vi "element A-D.vi"(8 "error in (no error)":errorcluster) -> (0 "error out":errorcluster, 3 "max(x,y)":i64)   [LabVIEW 2020, in "Settings.lvlib"]
uses:
  Settings.lvlib
  <vilib>/drjdpowell/SQLite Library/SQL Connection/Open (path).vi
  <vilib>/drjdpowell/SQLite Library/SQL Connection/Open (string).vi
  <vilib>/AdvancedString/Path To Command Line String.vi
  <vilib>/drjdpowell/SQLite Library/SQL Connection/Execute SQL (1D Integer results).vi
  <vilib>/drjdpowell/SQLite Library/SQL Connection/Connection.lvclass
  <vilib>/drjdpowell/SQLite Library/SQLite.lvlib
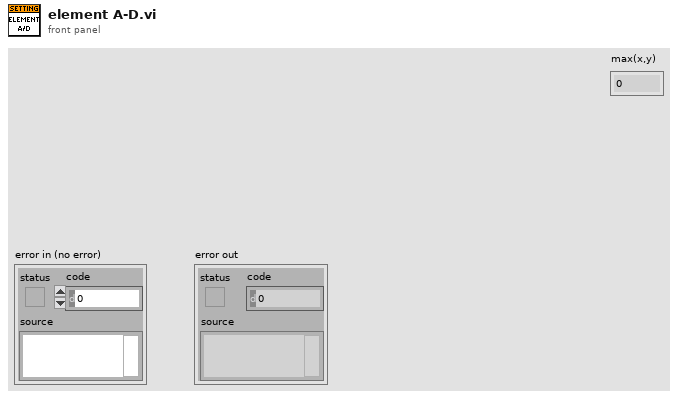
[diagram p1: front panel]
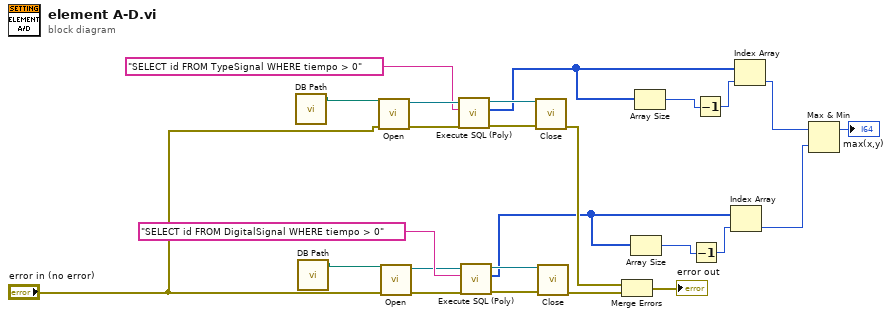
[diagram p0: block diagram]
diagram:
  n1 = call "DB Path.vi"() -> ("DB path"=w20:path)  [unwired: 11 in]
  n2 = call "DB Path.vi"() -> ("DB path"=w18:path)  [unwired: 11 in]
  n3 = call-poly <vilib>:"Open.vi"("error in (no error)"="error in (no error)", "db file"=w20) -> ("error out"=w24:errorcluster, "SQLite Connection"=w23:refnum<class "Connection.lvclass">)  [unwired: 8 in]
  n4 = call-poly <vilib>:"Open.vi"("error in (no error)"="error in (no error)", "db file"=w18) -> ("error out"=w13:errorcluster, "SQLite Connection"=w14:refnum<class "Connection.lvclass">)  [unwired: 8 in]
  n5 = call-poly <vilib>:"Execute SQL (Poly).vi"("error in (no error)"=w24, "SQL"="SELECT id FROM TypeSignal WHERE tiempo > 0", "SQLite Connection in"=w23) -> ("error out"=w21:errorcluster, "Result Set"=w9:i64[], "SQLite Connection"=w22:refnum<class "Connection.lvclass">)  [unwired: 5 in, 1 out]
  n6 = call-poly <vilib>:"Execute SQL (Poly).vi"("error in (no error)"=w13, "SQL"="SELECT id FROM DigitalSignal WHERE tiempo > 0", "SQLite Connection in"=w14) -> ("error out"=w16:errorcluster, "Result Set"=w4:i64[], "SQLite Connection"=w15:refnum<class "Connection.lvclass">)  [unwired: 5 in, 1 out]
  n7 = call-dynamic "Close.vi"("error in (no error)"=w21, "SQLite Connection in"=w22) -> ("error out"=w10:errorcluster)  [unwired: 9 in]
  n8 = call-dynamic "Close.vi"("error in (no error)"=w16, "SQLite Connection in"=w15) -> ("error out"=w25:errorcluster)  [unwired: 9 in]
  n9 = Merge Errors(w10, w25) -> (→"error out":errorcluster)
  n10 = Array Size(array=w4) -> (size(s)=w6:i32)
  n11 = Array Size(array=w9) -> (size(s)=w8:i32)
  n12 = Decrement(x=w6) -> (x-1=w5:i32)
  n13 = Decrement(x=w8) -> (x-1=w7:i32)
  n14 = Index Array(array=w4, index=w5) -> (element=w2:i64)
  n15 = Index Array(array=w9, index=w7) -> (element=w3:i64)
  n16 = Max & Min(x=w3, y=w2) -> (max(x,y)=→"max(x,y)":i64)  [unwired: 1 out]
